vi "TeddingtonClient.vi"() -> (0 "Time Of Value (s)":dbl format="%#.1f", 1 "Error":bool, 2 "Sea level Pressure String/mBar":dbl)   [LabVIEW 2016]
panel:
  out "Time Stamp GMT":timestamp
  out "data out":string
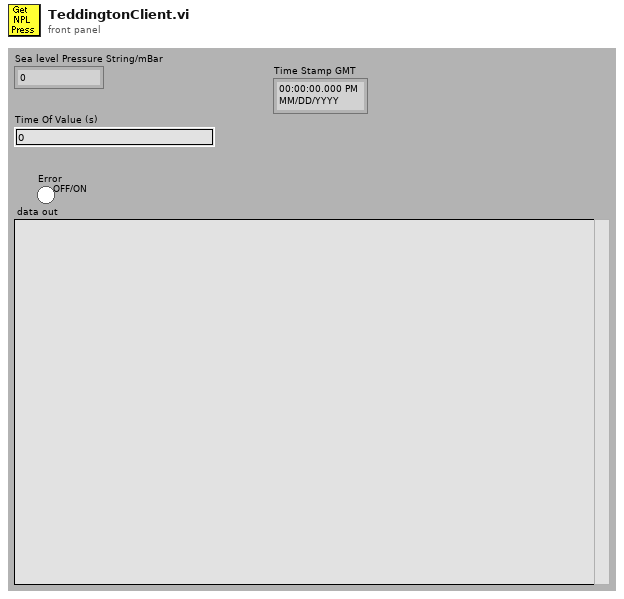
[diagram p1: front panel]
types:
  T1 = enum16{"Standard", "Buffered", "CRLF", "Immediate"}
  T2 = cluster{"second":i32, "minute":i32, "hour":i32, "day of month":i32, "month":i32, "year":i32, "day of week":i32, "day of year":i32, "is DST":i32}
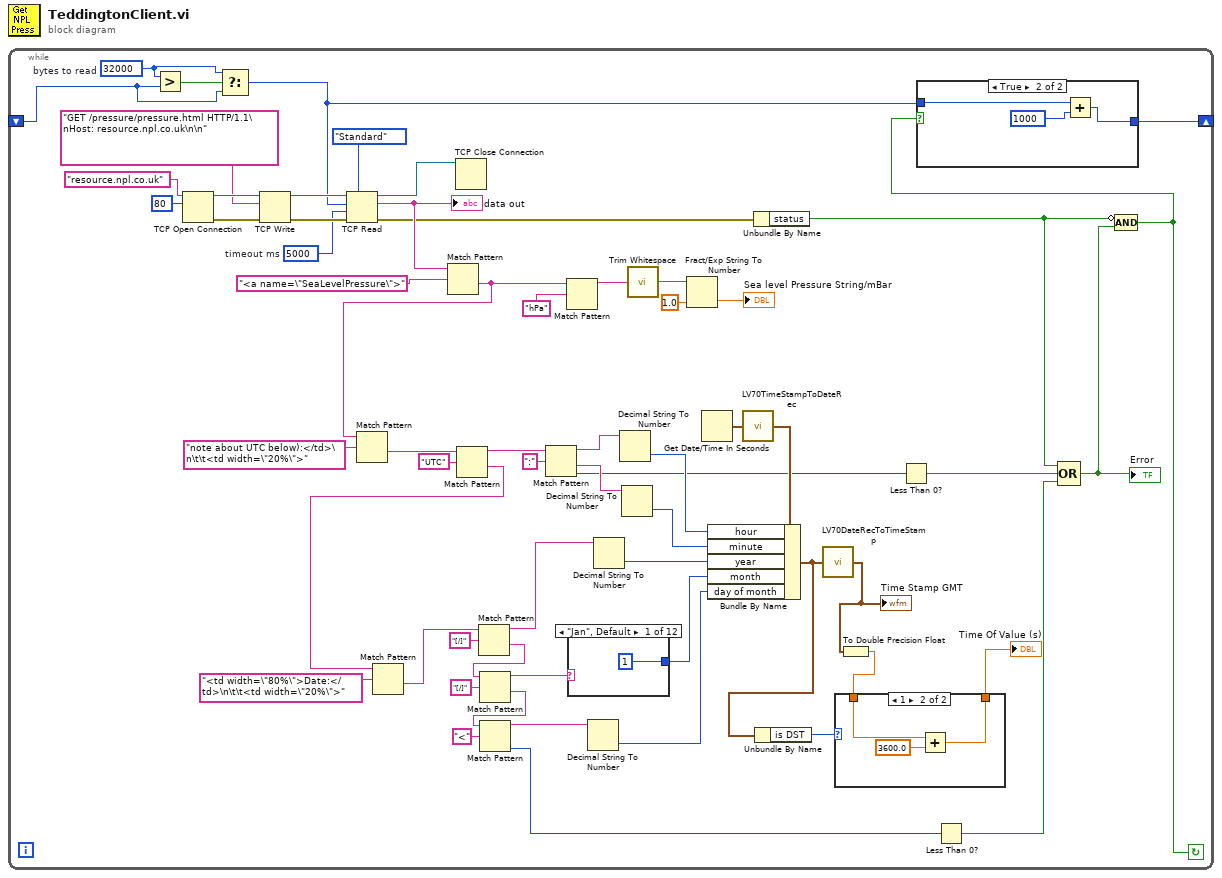
[diagram p0: block diagram]
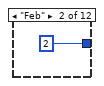
[diagram p4: hidden frame]
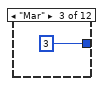
[diagram p5: hidden frame]
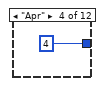
[diagram p6: hidden frame]
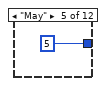
[diagram p7: hidden frame]
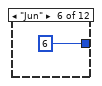
[diagram p8: hidden frame]
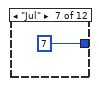
[diagram p9: hidden frame]
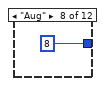
[diagram p10: hidden frame]
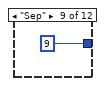
[diagram p11: hidden frame]
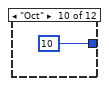
[diagram p12: hidden frame]
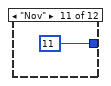
[diagram p13: hidden frame]
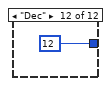
[diagram p14: hidden frame]
diagram:
  n1 = while {
    shift-right: [w3] -> _
    shift-left: _ -> [w7]
    stop <- w2 continue-if-true
    w13 = 5000  # timeout ms
    w8 = 32000  # bytes to read
    n2 = Greater?(x=w8, y=w7) -> (0:w9:bool)
    n3 = TCP Open Connection(address="resource.npl.co.uk", remote port or service name=u16 80 ("remote port")) -> (connection ID=w59:refnum<k5>, error out=w57:errorcluster)  [unwired: 1 in, 2 out]
    n4 = Select(t=w8, s=w9, f=w7) -> (s? t:f=w4:i32)
    n5 = TCP Write(connection ID=w59, data in="GET /pressure/pressure.html HTTP/1.1\nHost: resource.npl.co.uk\n\n", error in (no error)=w57) -> (connection ID out=w54:refnum<k5>, error out=w56:errorcluster)  [unwired: 2 out]
    n6 = TCP Read(connection ID=w54, bytes to read=w4, error in (no error)=w56, 7:T1."Standard" ("mode (standard)"), 9:w13) -> (connection ID out=w55:refnum<k5>, data out=w15:string, error out=w1:errorcluster)
    "data out" <- w15
    n7 = Match Pattern(string=w15, regular expression="<a name=\"SeaLevelPressure\">") -> (after substring=w16:string)  [unwired: 4 out]
    n8 = Match Pattern(string=w16, regular expression="note about UTC below):</td>\n\t\t<td width=\"20%\">") -> (after substring=w48:string)  [unwired: 4 out]
    n9 = TCP Close Connection(connection ID=w55) -> ()  [unwired: 1 in, 3 out]
    n10 = Match Pattern(string=w48, regular expression="UTC") -> (before substring=w43:string, after substring=w29:string)  [unwired: 3 out]
    n11 = Match Pattern(string=w29, regular expression="<td width=\"80%\">Date:</td>\n\t\t<td width=\"20%\">") -> (after substring=w41:string)  [unwired: 4 out]
    n12 = Match Pattern(string=w41, regular expression="[/]") -> (before substring=w37:string, after substring=w36:string)  [unwired: 3 out]
    n13 = Match Pattern(string=w36, regular expression="[/]") -> (before substring=w34:string, after substring=w35:string)  [unwired: 3 out]
    n14 = Match Pattern(string=w35, regular expression="<") -> (before substring=w32:string, offset past match=w23:i32)  [unwired: 3 out]
    n15 = Match Pattern(string=w43, regular expression=":") -> (before substring=w47:string, after substring=w46:string, offset past match=w22:i32)  [unwired: 2 out]
    n16 = Match Pattern(string=w16, regular expression="hPa") -> (before substring=w11:string)  [unwired: 4 out]
    n17 = case shown="\"Jan\", Default" w34 {
      tunnel: [1 ("month") 2 ("month") 3 ("month") 4 ("month") 5 ("month") 6 ("month") 7 ("month") 8 ("month") 9 ("month") 10 ("month") 11 ("month") 12 ("month")] -> w33
      frame "Jan", Default {
      }
      frame "Feb" {
      }
      frame "Mar" {
      }
      frame "Apr" {
      }
      frame "May" {
      }
      frame "Jun" {
      }
      frame "Jul" {
      }
      frame "Aug" {
      }
      frame "Sep" {
      }
      frame "Oct" {
      }
      frame "Nov" {
      }
      frame "Dec" {
      }
    }
    n18 = Decimal String To Number(string=w32) -> (number=w31:i32)  [unwired: 3 out]
    n19 = Decimal String To Number(string=w37) -> (number=w38:i32)  [unwired: 3 out]
    n20 = Decimal String To Number(string=w47) -> (number=w44:i32)  [unwired: 3 out]
    n21 = Decimal String To Number(string=w46) -> (number=w45:i32)  [unwired: 3 out]
    n22 = call <vilib>:"Trim Whitespace.vi"("string"=w11) -> ("trimmed string"=w19:string)  [unwired: 1 in]
    n23 = Fract/Exp String To Number(string=w19, default (0 dbl)=1.0 ("default (0 DBL)")) -> (number=→"Sea level Pressure String/mBar":dbl)  [unwired: 3 out]
    n24 = Get Date/Time In Seconds() -> (seconds since 1Jan1904=w12:timestamp)
    n25 = call <vilib>:"LV70TimeStampToDateRec.vi"("time stamp"=w12) -> ("date time rec"=w28:T2)
    n26 = Bundle By Name(cluster=w28, "hour"=w44, "minute"=w45, "year"=w38, "month"=w33, "day of month"=w31) -> (w26:T2)
    n27 = Unbundle By Name(w1) -> ("status"=w6:bool)
    n28 = Unbundle By Name(w26) -> ("is DST"=w25:i32)
    n29 = call <vilib>:"LV70DateRecToTimeStamp.vi"("date time rec"=w26) -> ("Time Stamp"=w27:timestamp)
    "Time Stamp GMT" <- w27
    n30 = To Double Precision Float(number=w27) -> (double precision float=w24:dbl)
    n31 = case shown="1" w25 {
      tunnel: w24 -> [w66 w69]
      tunnel: [w66 w67] -> w14
      frame 0, Default {
      }
      frame 1 {
        n32 = Add(x=w69, y=3600.0) -> (x+y=w67:dbl)
      }
    }
    "Time Of Value (s)" <- w14
    n33 = Less Than 0?(x=w22) -> (x < 0?=w17:bool)
    n34 = Less Than 0?(x=w23) -> (x < 0?=w18:bool)
    n35 = Compound Arithmetic op=OR(w6, w17, w18) -> (w5:bool)
    "Error" <- w5
    n36 = Compound Arithmetic op=AND(invert w6, w5) -> (w2:bool)
    n37 = case shown="True" w2 {
      tunnel: w4 -> [w62 w64]
      tunnel: [w62 w63] -> w3
      frame False {
      }
      frame True {
        n38 = Add(x=w64, y=1000 ("x")) -> (x+y=w63:i32)
      }
    }
  }
